vi "delete tag.vi"(8 "error in":errorcluster, 10 "tag name":string, 11 "file io module configuration in":refnum<class "file io module configuration.lvclass">) -> (0 "error out":errorcluster, 2 "deleted channels":refnum<class "TBM channel.lvclass">[](array[class]), 3 "file io module configuration out":refnum<class "file io module configuration.lvclass">)   [LabVIEW 2013, in "file io module configuration.lvclass"]
uses:
  file io module configuration.lvclass
  <vilib>/NI/Tag Bus Module Framework/channel/TBM channel.lvclass
  file io module configuration.lvclass/file io module configuration.ctl
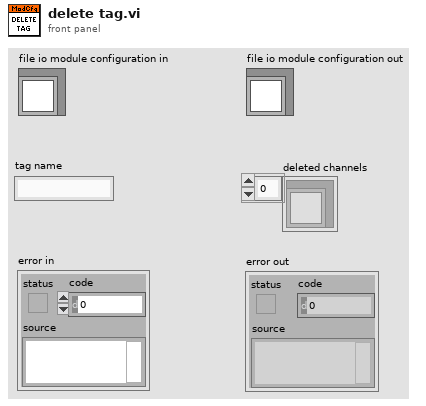
[diagram p1: front panel]
types:
  T1 = typedef "file io module configuration.lvclass/line configuration.ctl" = cluster{"name":string, "data type":T2, "channel":refnum<class "TBM channel.lvclass">}
  T2 = typedef "tag bus.lvlib/tag descriptor.lvclass/Data Type.ctl" = enum16{"Double", "Single", "I64", "I32", "I16", "I8", "U64", "U32", "U16", "U8", "Boolean", "String", "Array of Double", "Array of Single", "Array of I64", "Array of I32", "Array of I16", "Array of I8", "Array of U64", "Array of U32", "Array of U16", "Array of U8", "Array of Boolean", "Array of String"}
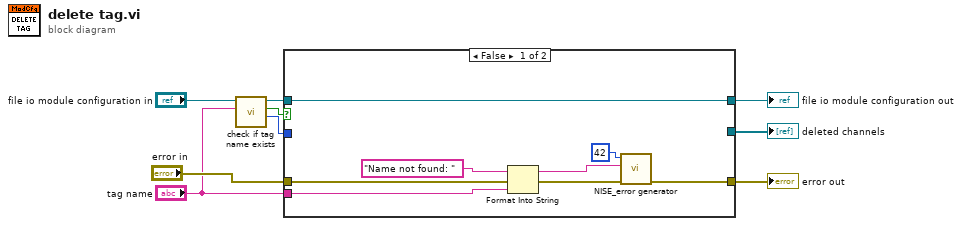
[diagram p0: block diagram]
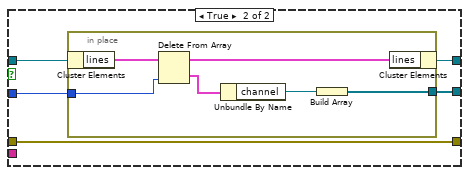
[diagram p2: hidden frame]
diagram:
  n1 = call "check if tag name exists.vi"("name to locate"="tag name", "file io module configuration in"="file io module configuration in") -> ("index"=w1:i32, "found?"=w3:bool, "file io module configuration out"=w2:refnum<class "file io module configuration.lvclass">)  [unwired: 6 in, 1 out]
  n2 = case shown="False" w3 {
    tunnel: [w16 w20] -> w8
    tunnel: "error in" -> [w17 w20]
    tunnel: [w11 w21] -> w6
    tunnel: w2 -> [w11 w22]
    tunnel: [_ w19] -> w5
    tunnel: w1 -> [_ w18]
    tunnel: "tag name" -> [w10 _]
    frame False {
      n3 = Format Into String(initial string="Name not found: " ("append error message"), error in=w17, w10) -> (resulting string=w12:string, error out=w14:errorcluster)  [unwired: 1 in]
      n4 = call <vilib>:"NISE_error generator.vi"("error in"=w14, "append error message"=w12, "error code (0)"=42) -> ("error out"=w16:errorcluster)  [unwired: 6 in]
    }
    frame True {
      n5 = in-place {
        in-place-border: [w24] -> w19
        in-place-border: w18 -> [w26]
        n6 = in-place-cluster #1(w22) -> ("lines"=w28:T1[])
        n7 = Delete From Array(array=w28, index=w26) -> (deleted portion=w25:T1, array with subset deleted=w27:T1[])  [unwired: 1 in]
        n8 = Unbundle By Name(w25) -> ("channel"=w23:refnum<class "TBM channel.lvclass">)
        n9 = Build Array(w23) -> (w24:refnum<class "TBM channel.lvclass">[])
        n10 = in-place-cluster #1("lines"=w27) -> (w21:refnum<class "file io module configuration.lvclass">)
      }
    }
  }
  "error out" <- w8
  "file io module configuration out" <- w6
  "deleted channels" <- w5
